vi "Update User Plugin.vi"(8 "error in (no error)":errorcluster, 10 "Plugin Reference":refnum<class "DCM-DSI.lvclass">, 11 "DSI Reference":refnum<class "DCM-DSI.lvclass">) -> (0 "error out":errorcluster, 2 "Plugin Reference":refnum<class "DCM-DSI.lvclass">, 3 "DSI Reference":refnum<class "DCM-DSI.lvclass">)   [LabVIEW 2016, in "DCM-DSI.lvclass"]
uses:
  DCM-DSI.lvclass
  DCM-DSI.lvclass/DCM-DSI.ctl
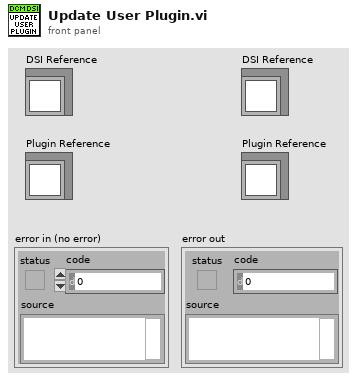
[diagram p1: front panel]
types:
  T1 = cluster{"DCM Ref":refnum<class "DCM - RT.lvclass">, "ExpansionRIO Ref":refnum<data-value>, "DiffIO Results":refnum<data-value>, "DiffIO State":refnum<data-value>, "DiffIO Setup":refnum<data-value>, "EPTx Data":refnum<data-value>, "ESTTL Setup":refnum<data-value>, "Knock Results":refnum<data-value>, "HH Config":refnum<data-value>, "HH Command":refnum<data-value>, "HH Scope Data":refnum<data-value>, "HH Scope Ctr":refnum<data-value>, "HH Status":refnum<data-value>, "DI-A Command":refnum<data-value>, "DI-B Command":refnum<data-value>, "DI-A Profiles":refnum<data-value>, "DI-B Profiles":refnum<data-value>, "DI Scope Data":refnum<data-value>, "DI Scope dt [s]":refnum<data-value>, "DI Scope Ctr":refnum<data-value>, "Pump-A Command":refnum<data-value>, "Pump-B Command":refnum<data-value>, "Skip Fire Setup":refnum<data-value>, "System State":refnum<data-value>}
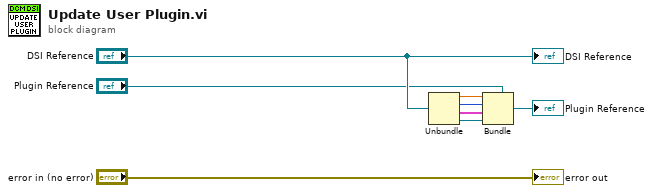
[diagram p0: block diagram]
diagram:
  n1 = Unbundle("DSI Reference") -> (w7:dbl, w6:i32, w5:T1, w4:refnum<data-value>)
  n2 = Bundle(cluster="Plugin Reference", w7, w6, w5, w4) -> (→"Plugin Reference":refnum<class "DCM-DSI.lvclass">)
  "error out" <- "error in (no error)"
  "DSI Reference" <- "DSI Reference"
